vi "bitrate n2e.vi"(1 "number":u16 format="%0d") -> (0 "enum":T1=enum."RATE_1Mbps")   [LabVIEW 2024, in "atsj peakcan basic.lvlib"]
uses:
  bitrate.ctl
  atsj peakcan basic.lvlib
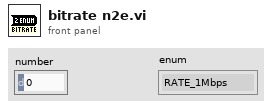
[diagram p1: front panel]
types:
  T1 = typedef "atsj peakcan basic.lvlib/bitrate.ctl" = enum16{"RATE_UNSUPPORTED", "RATE_1Mbps", "RATE_800kbps", "RATE_500kbps", "RATE_250kbps", "RATE_125kbps", "RATE_100kbps", "RATE_95kbps", "RATE_83kbps", "RATE_50kbps", "RATE_47kbps", "RATE_33kbps", "RATE_20kbps", "RATE_10kbps", "RATE_5kbps"}
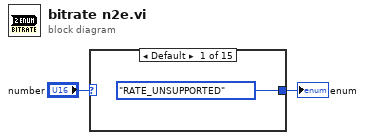
[diagram p0: block diagram]
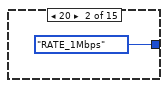
[diagram p2: hidden frame]
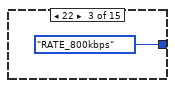
[diagram p3: hidden frame]
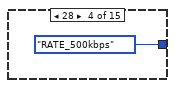
[diagram p4: hidden frame]
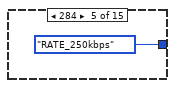
[diagram p5: hidden frame]
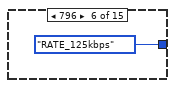
[diagram p6: hidden frame]
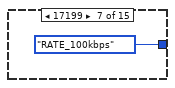
[diagram p7: hidden frame]
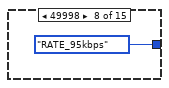
[diagram p8: hidden frame]
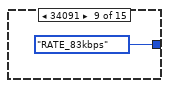
[diagram p9: hidden frame]
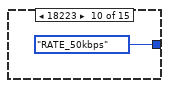
[diagram p10: hidden frame]
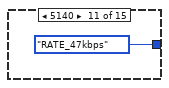
[diagram p11: hidden frame]
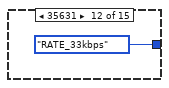
[diagram p12: hidden frame]
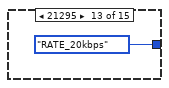
[diagram p13: hidden frame]
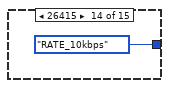
[diagram p14: hidden frame]
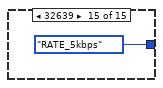
[diagram p15: hidden frame]
diagram:
  n1 = case shown="Default" "number" {
    tunnel: [bitrate."RATE_UNSUPPORTED" bitrate."RATE_1Mbps" bitrate."RATE_800kbps" bitrate."RATE_500kbps" bitrate."RATE_250kbps" bitrate."RATE_125kbps" bitrate."RATE_100kbps" bitrate."RATE_95kbps" bitrate."RATE_83kbps" bitrate."RATE_50kbps" bitrate."RATE_47kbps" bitrate."RATE_33kbps" bitrate."RATE_20kbps" bitrate."RATE_10kbps" bitrate."RATE_5kbps"] -> w1
    frame Default {
    }
    frame 20 {
    }
    frame 22 {
    }
    frame 28 {
    }
    frame 284 {
    }
    frame 796 {
    }
    frame 17199 {
    }
    frame 49998 {
    }
    frame 34091 {
    }
    frame 18223 {
    }
    frame 5140 {
    }
    frame 35631 {
    }
    frame 21295 {
    }
    frame 26415 {
    }
    frame 32639 {
    }
  }
  "enum" <- w1
